vi "buildFrame.vi"(7 "Data":string, 8 "error in":errorcluster, 9 "Sensor Selector":string, 10 "Dictionary Selector":string, 11 "Dictionary ID":string) -> (0 "error out":errorcluster, 1 "H2F Checksum":string, 2 "Frame w/o crc":string, 3 "H2F Frame":string)   [LabVIEW 2018]
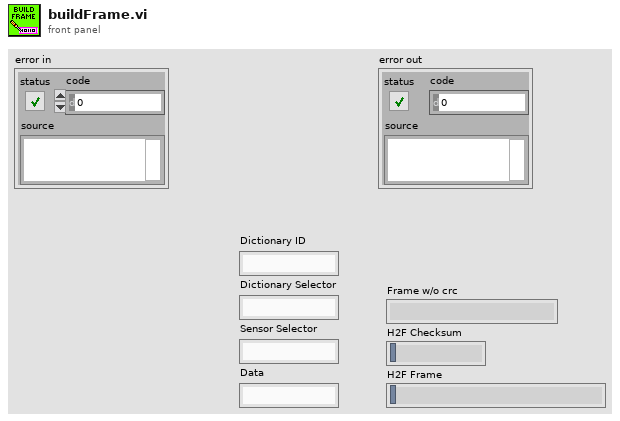
[diagram p1: front panel]
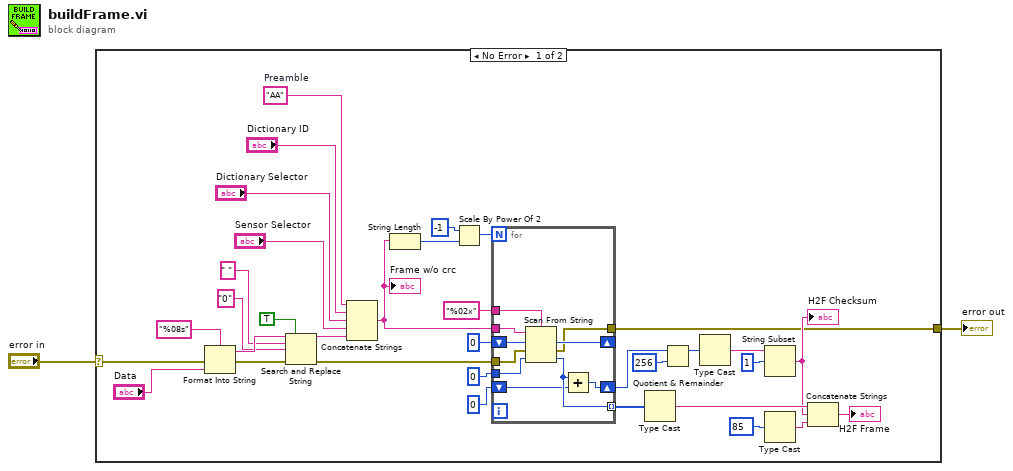
[diagram p0: block diagram]
diagram:
  n1 = case shown="No Error" "error in" {
    selector: "error in" -> [w6 w47]
    tunnel: [w3 w47] -> w1
    frame No Error {
      w34 = "AA"  # Preamble
      n2 = Format Into String(format string="%08s", error in=w6, "Data") -> (resulting string=w11:string, error out=w5:errorcluster)  [unwired: 1 in]
      n3 = Search and Replace String(replace all?=TRUE ("replace all? (F)"), input string=w11, search string=" ", replace string="0" ("replace string (\"\")"), error in=w5) -> (result string=w7:string, error out=w4:errorcluster)  [unwired: 3 in, 2 out]
      n4 = Concatenate Strings(w34, "Dictionary ID", "Dictionary Selector", "Sensor Selector", w7) -> (w29:string)
      "Frame w/o crc" <- w29
      n5 = String Length(string=w29) -> (length=w32:i32)
      n6 = Scale By Power Of 2(n=i16 -1, x=w32) -> (x*2^n=w30:i32)
      n7 = for {
        N: w30 -> [_]
        tunnel: w29 -> [w46]
        tunnel: "%02x" -> [w45]
        shift-right: [w44] -> _
        shift-left: u32 0 -> [w43]
        tunnel: u8 0 -> [w42]
        tunnel: [w41] -> w26 mode=indexing
        shift-right: [w40] -> w25
        shift-left: u8 0 -> [w39]
        tunnel: w4 -> [w38]
        tunnel: [w37] -> w3
        n8 = Scan From String(format string=w45, input string=w46, initial scan location=w43, error in=w38, default 1=w42) -> (offset past scan=w44:u32, error out=w37:errorcluster, output 1=w41:u8)  [unwired: 1 out]
        n9 = Add(x=w41, y=w39) -> (x+y=w40:u8)
      }
      n10 = Type Cast(x=w26) -> (*(type *) &x=w23:string)  [unwired: 1 in]
      n11 = Quotient & Remainder(x=w25, y=u16 256) -> (x-y*floor(x/y)=w18:u16)  [unwired: 1 out]
      n12 = Type Cast(x=w18) -> (*(type *) &x=w17:string)  [unwired: 1 in]
      n13 = String Subset(string=w17, offset (0)=1) -> (substring=w16:string)  [unwired: 1 in]
      "H2F Checksum" <- w16
      n14 = Type Cast(x=u8 85) -> (*(type *) &x=w21:string)  [unwired: 1 in]
      n15 = Concatenate Strings(w23, w16, w21) -> (→"H2F Frame":string)
    }
    frame Error {
    }
  }
  "error out" <- w1
